vi "FileIO_CreateDirectory.vi"(0 "Base Path":path, 5 "Directory Name":string, 11 "Error In":errorcluster) -> (4 "File Path Control":path, 15 "Error Out":errorcluster)   [LabVIEW 2023]
doc: "This VI will create a folder/diectory to desired path with desired name."
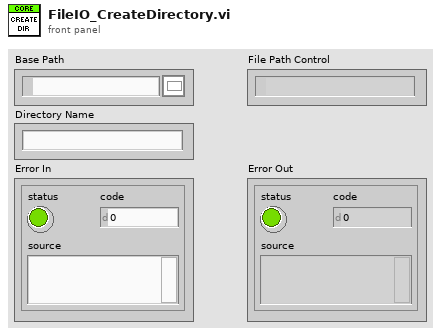
[diagram p1: front panel]
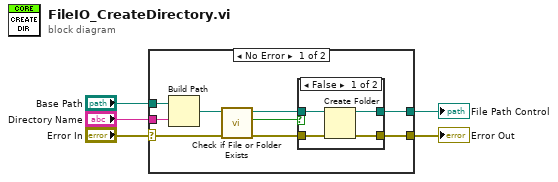
[diagram p0: block diagram]
diagram:
  n1 = case shown="No Error" "Error In" {
    selector: "Error In" -> [w10 w21]
    tunnel: "Directory Name" -> [w14 _]
    tunnel: "Base Path" -> [w13 _]
    tunnel: [w12 w21] -> w3
    tunnel: [w11 _] -> w1
    frame No Error {
      n2 = Build Path(base path=w13, name or relative path=w14) -> (appended path=w8:path)
      n3 = call <vilib>:"Check if File or Folder Exists.vi"("error in (no error)"=w10, "path"=w8) -> ("error out"=w9:errorcluster, "file or folder exists?"=w7:bool, "dup path"=w6:path)  [unwired: 7 in]
      n4 = case shown="False" w7 {
        tunnel: [w18 w19] -> w12
        tunnel: [w17 w20] -> w11
        tunnel: w9 -> [w16 w19]
        tunnel: w6 -> [w15 w20]
        frame False {
          n5 = Create Folder(path (use dialog)=w15, error in=w16) -> (created path=w17:path, error out=w18:errorcluster)  [unwired: 1 in, 1 out]
        }
        frame True {
        }
      }
    }
    frame Error {
    }
  }
  "Error Out" <- w3
  "File Path Control" <- w1
